vi "CPU_PC_inc.vi"(11 "registers":T1={"A"=0, "X"=0, "Y"=0, "SP"=253, "PC"=0, "P"=36} {"P" format="%08b"; "PC" format="%04x"; "SP" format="%02x"; "Y" format="%02x"; "X" format="%02x"; "A" format="%02x"}) -> (3 "registers":T1={"A"=0, "X"=0, "Y"=0, "SP"=253, "PC"=0, "P"=36} {"P" format="%08b"; "PC" format="%04x"; "SP" format="%02x"; "Y" format="%02x"; "X" format="%02x"; "A" format="%02x"})   [LabVIEW 2018]
uses:
  CPU_registers.ctl
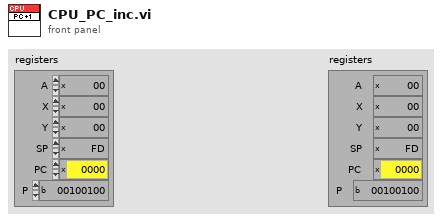
[diagram p1: front panel]
types:
  T1 = typedef "CPU_registers.ctl" = cluster{"A":u8, "X":u8, "Y":u8, "SP":u8, "PC":u16, "P":u8}
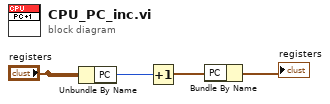
[diagram p0: block diagram]
diagram:
  n1 = Unbundle By Name("registers") -> ("PC"=w4:u16)
  n2 = Increment(x=w4) -> (x+1=w2:u16)
  n3 = Bundle By Name(cluster="registers", "PC"=w2) -> (→"registers":T1)
